vi "Follow 1D Motion Profile for Turning.vi"(4 "PID gains":T20 {"derivative time (Td, min)" format="%.3f"; "integral time (Ti, min)" format="%.3f"; "proportional gain (Kc)" format="%.3f"}, 6 "Period (s)":dbl=0.005, 7 "output range":cluster{"output high":dbl, "output low":dbl}={"output high"=1.0, "output low"=-1.0} {"output low" format="%.2f"; "output high" format="%.2f"}, 8 "Ka":dbl, 9 "Kv":dbl, 10 "Profile":T21, 11 "auton ref":T1={"Starting Pos"=0, "Defence"=enum."Chivel De Fris", "Drivetrain"={"DevStatus"={"status"=FALSE, "code"=0, "source"=""}, "Motors[]"=[], "Square Inputs"=FALSE, "Max Output"=1.0}, "State"=enum."Drive to Outerworks", "Encoder Right"={"DevStatus"={"status"=FALSE, "code"=0, "source"=""}, "EncoderIndex"=enum."Invalid", "CounterIndex"=enum."Invalid", "DistancePerCount"=1.0, "Decoding Type"=enum."4x"}, "Encoder Left"={"DevStatus"={"status"=FALSE, "code"=0, "source"=""}, "EncoderIndex"=enum."Invalid", "CounterIndex"=enum."Invalid", "DistancePerCount"=1.0, "Decoding Type"=enum."4x"}, "Line Sensor"={"DevStatus"={"status"=FALSE, "code"=0, "source"=""}, "DIO Channel"=enum."Invalid", "CntIndex"=enum."Invalid", "Normally Closed"=FALSE}, "navX"={"Interface"={"Protocol"=enum."SERIAL", "Update Rate (4Hz-60Hz)"=4, "navX Open TypeDef"=variant}, "Notify Packet"=refnum, "Loop VI Refnum"=refnum, "Ready to Close Occurrence Refnum"=refnum}, "Front Arm"={"DevStatus"={"status"=FALSE, "code"=0, "source"=""}, "Analog Channel"=enum."Invalid", "Invert Output"=FALSE}, "Start Time"=0, "State Vars"=variant} {"navX"."Interface"."Update Rate (4Hz-60Hz)" min=4 max=60 step=1}) -> ()   [LabVIEW 2016]
uses:
  <vilib>/Platform/TimedLoop/XDataNode/XDataNode.xnode
  <vilib>/Platform/TimedLoop/XDataNode/nitl_modes.ctl
  <vilib>/Platform/TimedLoop/XDataNode/XDNodeRunTimeDep.lvlib
  <vilib>/Platform/TimedLoop/XDataNode/wakeup.ctl
  <vilib>/Platform/TimedLoop/XDataNode/timing_clust.ctl
  <vilib>/addons/control/pid/NI_PID_pid.lvlib
  <vilib>/addons/control/pid/pid.llb/PID (DBL).vi
  Robot Global Data.vi
  Typedef/Motion Profile.ctl
  NavX/TypeDefs/Z900_navX_ProtocolTypeDef.ctl
  NavX/TypeDefs/Z900_navX_ActionTypeDef.ctl
  NavX/TypeDefs/Z900_navX_NotifyPacketTypeDef.ctl
  NavX/TypeDefs/Z900_navX_DeviceTypeDef.ctl
  <vilib>/Rock Robotics/SystemInterfaces/DIO/FPGA_DIOChannel.ctl
  <vilib>/Rock Robotics/SystemInterfaces/Counter/FPGA_CounterCtrSystemIndex.ctl
  <vilib>/Rock Robotics/WPI/Switch/WPI_SwitchDevRef.ctl
  <vilib>/Rock Robotics/SystemInterfaces/Encoder/FPGA_EncoderIdx.ctl
  <vilib>/Rock Robotics/WPI/Encoder/WPI_EncoderType.ctl
  <vilib>/Rock Robotics/WPI/Encoder/WPI_EncoderDevRef.ctl
  Typedef/MainStates.ctl
  <vilib>/Rock Robotics/SystemInterfaces/DIO/FPGA_DIOPWMChannel.ctl
  <vilib>/Rock Robotics/WPI/PWM/WPI_PWMDeadband.ctl
  <vilib>/Rock Robotics/WPI/MotorControl/WPI_MotorControlType.ctl
  <vilib>/Rock Robotics/WPI/MotorControl/WPI_MotorControlDeviceRef.ctl
  <vilib>/Rock Robotics/WPI/RobotDrive/WPI_RobotDriveDevRef.ctl
  Typedef/Defences.ctl
  Typedef/AutonRefType.ctl
  <vilib>/Rock Robotics/SystemInterfaces/AI/FPGA_AIChannel.ctl
  <vilib>/Rock Robotics/WPI/Potentiometer/WPI_PotentiometerDevRef.ctl
panel:
  in  "Eliminate Deadband":bool=TRUE
  out "Waveform Chart":T19(graph)
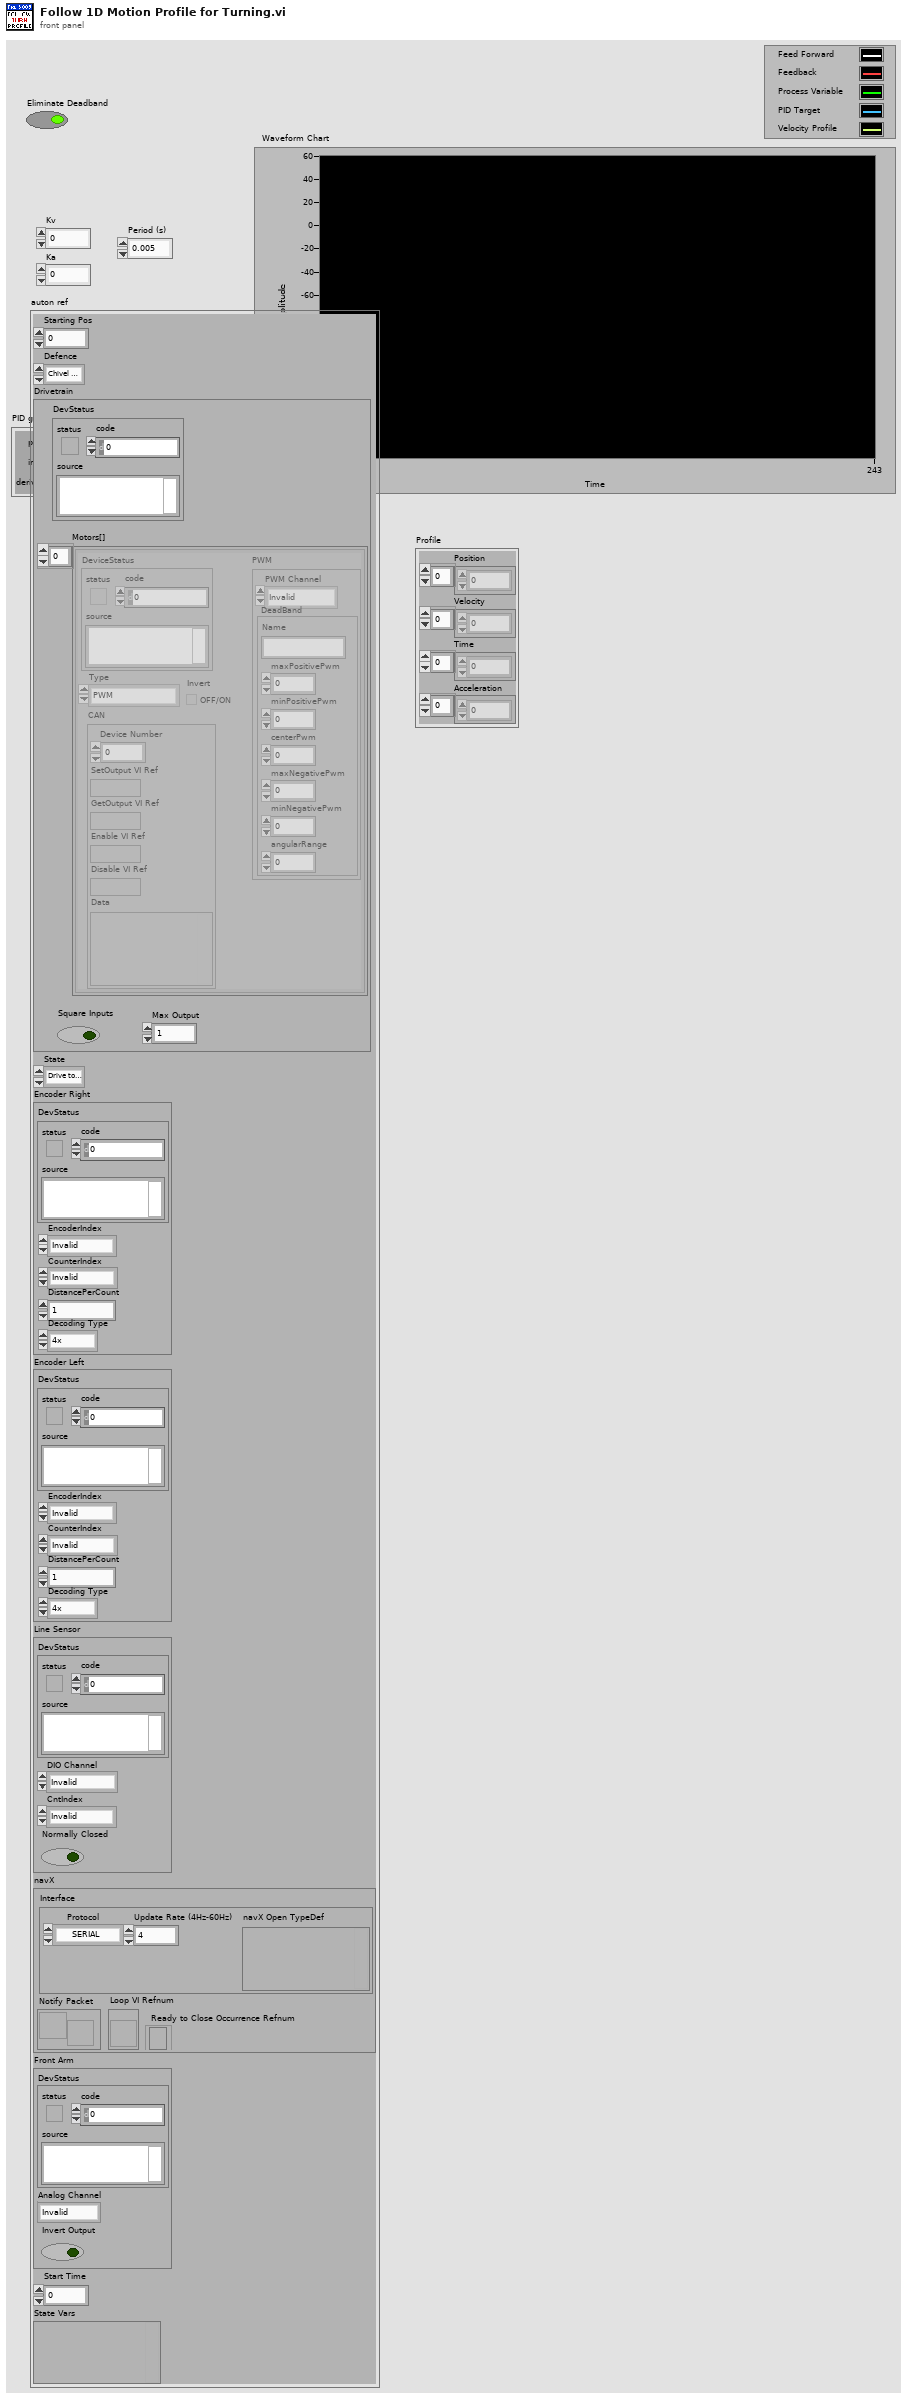
[diagram p1: front panel]
types:
  T1 = typedef "AutonRefType.ctl" = cluster{"Starting Pos":u32, "Defence":T2, "Drivetrain":T3, "State":T8, "Encoder Right":T9, "Encoder Left":T9, "Line Sensor":T13, "navX":T15, "Front Arm":T17, "Start Time":u32, "State Vars":variant}
  T2 = typedef "Defences.ctl" = enum16{"Low Bar", "Chivel De Fris", "Sally Port", "Portcullis", "Draw Bridge", "Moat", "Rough Terrain", "Ramparts", "Rock Wall"}
  T3 = typedef "WPI_RobotDriveDevRef.ctl" = cluster{"DevStatus":errorcluster, "Motors[]":T4[], "Square Inputs":bool, "Max Output":dbl}
  T4 = typedef "WPI_MotorControlDeviceRef.ctl" = cluster{"DeviceStatus":errorcluster, "Type":T5, "PWM":cluster{"PWM Channel":T6, "DeadBand":T7}, "CAN":cluster{"Device Number":u8, "SetOutput VI Ref":variant, "GetOutput VI Ref":variant, "Enable VI Ref":variant, "Disable VI Ref":variant, "Data":variant}, "Invert":bool}
  T5 = typedef "WPI_MotorControlType.ctl" = enum16{"PWM", "CAN"}
  T6 = typedef "FPGA_DIOPWMChannel.ctl" = enum8{"PWM 0", "PWM 1", "PWM 2", "PWM 3", "PWM 4", "PWM 5", "PWM 6", "PWM 7", "PWM 8", "PWM 9", "PWM MXP 0", "PWM MXP 1", "PWM MXP 2", "PWM MXP 3", "PWM MXP 4", "PWM MXP 5", "PWM MXP 6", "PWM MXP 7", "PWM MXP 8", "PWM MXP 9", "Invalid"}
  T7 = typedef "WPI_PWMDeadband.ctl" = cluster{"Name":string, "maxPositivePwm":i32, "minPositivePwm":i32, "centerPwm":i32, "maxNegativePwm":i32, "minNegativePwm":i32, "angularRange":u16}
  T8 = typedef "MainStates.ctl" = enum16{"Drive to Outerworks", "Cross Defence", "Align to Line", "Turn to Goal", "Find Position", "Find Distance", "Drive to Scoring Location", "Score Low Goal", "SquareToField", "Hit Driver Station Wall", "Drive Back to Position", "CDF", "Cleanup", "_TEST_Profile", "_TEST_TurnProfile", "_TEST_Impulse", "Error"}
  T9 = typedef "WPI_EncoderDevRef.ctl" = cluster{"DevStatus":errorcluster, "EncoderIndex":T10, "CounterIndex":T11, "DistancePerCount":dbl, "Decoding Type":T12}
  T10 = typedef "FPGA_EncoderIdx.ctl" = enum8{"Enc 0", "Enc 1", "Enc 2", "Enc 3", "Enc 4", "Enc 5", "Enc 6", "Enc 7", "Invalid"}
  T11 = typedef "FPGA_CounterCtrSystemIndex.ctl" = enum8{"Ctr 0", "Ctr 1", "Ctr 2", "Ctr 3", "Ctr 4", "Ctr 5", "Ctr 6", "Ctr 7", "Invalid"}
  T12 = typedef "WPI_EncoderType.ctl" = enum16{"1x", "2x", "4x"}
  T13 = typedef "WPI_SwitchDevRef.ctl" = cluster{"DevStatus":errorcluster, "DIO Channel":T14, "CntIndex":T11, "Normally Closed":bool}
  T14 = typedef "FPGA_DIOChannel.ctl" = enum8{"DIO 0", "DIO 1", "DIO 2", "DIO 3", "DIO 4", "DIO 5", "DIO 6", "DIO 7", "DIO 8", "DIO 9", "DIO MXP 0", "DIO MXP 1", "DIO MXP 2", "DIO MXP 3", "DIO MXP 4", "DIO MXP 5", "DIO MXP 6", "DIO MXP 7", "DIO MXP 8", "DIO MXP 9", "DIO MXP 10", "DIO MXP 11", "DIO MXP 12", "DIO MXP 13", "DIO MXP 14", "DIO MXP 15", "SPI Port CS1", "SPI Port CS2", "SPI Port CS3", "SPI Port MISO", "SPI Port MOSI", "Invalid"}
  T15 = typedef "navX Library v2.lvlib/Z900_navX_DeviceTypeDef.ctl" = cluster{"Interface":cluster{"Protocol":T16, "Update Rate (4Hz-60Hz)":u8, "navX Open TypeDef":variant}, "Notify Packet":refnum<notifier>, "Loop VI Refnum":refnum<vi>, "Ready to Close Occurrence Refnum":refnum<k4>}
  T16 = typedef "navX Library v2.lvlib/Z900_navX_ProtocolTypeDef.ctl" = enum16{"SERIAL", "I2C", "SPI"}
  T17 = typedef "WPI_PotentiometerDevRef.ctl" = cluster{"DevStatus":errorcluster, "Analog Channel":T18, "Invert Output":bool}
  T18 = typedef "FPGA_AIChannel.ctl" = enum8{"AI 0", "AI 1", "AI 2", "AI 3", "AI MXP 0", "AI MXP 1", "AI MXP 2", "AI MXP 3", "Invalid"}
  T19 = cluster{dbl, "output":dbl, dbl, dbl, "Max Velocity":dbl}
  T20 = cluster{"proportional gain (Kc)":dbl, "integral time (Ti, min)":dbl, "derivative time (Td, min)":dbl}
  T21 = typedef "Motion Profile.ctl" = cluster{"Position":dbl[], "Velocity":dbl[], "Time":dbl[], "Acceleration":dbl[]}
  T22 = cluster{"Yaw":dbl, "Roll":dbl, "Pitch":dbl, "Heading":dbl, "Fused Heading":dbl}
  T23 = typedef "XDNodeRunTimeDep.lvlib/timing_clust.ctl" = cluster{"Expected End [f-1]":u64, "Actual End [f-1]":u64, "Finished Late? [f-1]":bool, "Expected End [i-1]":u64, "Actual End [i-1]":u64, "Finished Late? [i-1]":bool, "Expected Start [i]":u64, "Actual Start [i]":u64, "Expected Start [f]":u64, "Actual Start [f]":u64, "Source Name":string, "Structure Name":string, "Period":i64, "Deadline":i64, "Offset":i64, "Start":i64, "Priority":i32, "Timeout":i32, "Mode":T24, "Wakeup Reason":T25, "Error":errorcluster, "Source Type":string, "Secondary Source Type":string, "Global End Time":u64, "Global Start Time":u64, "Frame Duration":u64, "Iteration Duration":u64, "Assigned CPU":i32, "I/O Scan Engine Mode":u32}
  T24 = typedef "XDNodeRunTimeDep.lvlib/nitl_modes.ctl" = enum32{"No Change", "Process missed periods, maintain original phase", "Discard missed periods, maintain original phase", "Process missed periods, ignore original phase", "Discard missed periods, ignore original phase"}
  T25 = typedef "XDNodeRunTimeDep.lvlib/wakeup.ctl" = enum32{"Normal", "Aborted", "Asynchronous wakeup", "Timing source error", "Timed loop error", "Timeout"}
  T26 = cluster{dbl, "output":dbl, dbl, "Angle (rads)":dbl, "Max Velocity":dbl}
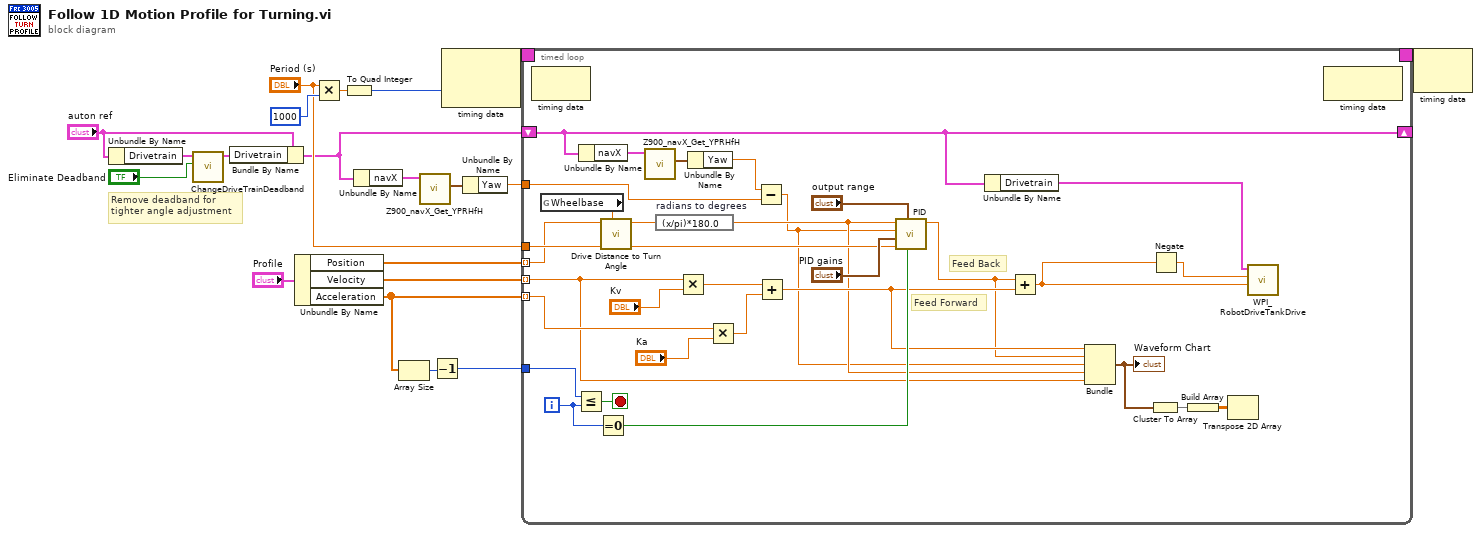
[diagram p0: block diagram]
diagram:
  # "Remove deadband for \ntighter angle adjustment"
  n1 = Unbundle By Name("auton ref") -> ("Drivetrain"=w5:T3)
  n2 = call "ChangeDriveTrainDeadband.vi"("Eliminate Deadband"="Eliminate Deadband", "Drivetrain in"=w5) -> ("Drivetrain out"=w2:T3)  [unwired: 9 in]
  n3 = Bundle By Name(cluster="auton ref", "Drivetrain"=w2) -> (w1:T1)
  n4 = Unbundle By Name("Profile") -> ("Position"=w17:dbl[], "Velocity"=w16:dbl[], "Acceleration"=w15:dbl[])
  n5 = Multiply(x="Period (s)", y=1000) -> (x*y=w11:dbl)
  n6 = To Quad Integer(1:w11) -> (0:w10:i64)
  n7 = Unbundle By Name(w1) -> ("navX"=w7:T15)
  n8 = Array Size(array=w15) -> (size(s)=w14:i32)
  n9 = call "Z900_navX_Get_YPRHfH.vi"("navX Device"=w7) -> ("YRPHfH"=w8:T22)  [unwired: 7 in, 3 out]
  n10 = Decrement(x=w14) -> (x-1=w13:i32)
  n11 = node-c288(w10) -> (w20:T23)  [unwired: 1 in]
  n12 = Unbundle By Name(w8) -> ("Yaw"=w6:dbl)
  n13 = timed-loop {
    timing: w20 -> [_]
    timing-out: [_] -> w19
    tunnel: w17 -> [w37] mode=indexing
    tunnel: w16 -> [w36] mode=indexing
    tunnel: w15 -> [w40] mode=indexing
    tunnel: w13 -> [w51]
    tunnel: "Period (s)" -> [w43]
    shift-right: [w35] -> _
    shift-left: w1 -> [w35]
    tunnel: w6 -> [w27]
    i -> [w42]
    stop <- w50 stop-if-true
    # "Feed Back"
    # "Feed Forward"
    n14 = node-c288() -> ()  [unwired: 1 in, 1 out]
    n15 = global read "Robot Global Data.vi" "Wheelbase"() -> (w30:dbl)
    n16 = Less Or Equal?(x=w51, y=w42) -> (x <= y?=w50:bool)
    n17 = Unbundle By Name(w35) -> ("navX"=w34:T15)
    n18 = Equal To 0?(x=w42) -> (x = 0?=w41:bool)
    n19 = call "Drive Distance to Turn Angle.vi"("Wheelbase (in)"=w30, "Distance (in)"=w37) -> ("Angle (rads)"=w31:dbl)  [unwired: 7 in]
    n20 = call "Z900_navX_Get_YPRHfH.vi"("navX Device"=w34) -> ("YRPHfH"=w33:T22)  [unwired: 7 in, 3 out]
    n21 = expression code="(x/pi)*180.0" "radians to degrees"(w31) -> (w29:dbl)
    n22 = Multiply(x=w36, y="Kv") -> (x*y=w47:dbl)
    n23 = Unbundle By Name(w33) -> ("Yaw"=w32:dbl)
    n24 = Multiply(x=w40, y="Ka") -> (x*y=w46:dbl)
    n25 = Subtract(x=w32, y=w27) -> (x-y=w28:dbl)
    n26 = Add(x=w47, y=w46) -> (x+y=w39:dbl)
    n27 = call-poly <vilib>:"PID.vi"("reinitialize? (F)"=w41, "output range"="output range", "dt (s)"=w43, "PID gains"="PID gains", "process variable"=w28, "setpoint"=w29) -> ("output"=w38:dbl)  [unwired: 4 in, 1 out]
    n28 = Unbundle By Name(w35) -> ("Drivetrain"=w21:T3)
    n29 = Add(x=w38, y=w39) -> (x+y=w26:dbl)
    n30 = Bundle(w39, "output"=w38, w28, "Angle (rads)"=w29, "Max Velocity"=w36) -> (w22:T26)  [unwired: 1 in]
    "Waveform Chart" <- w22
    n31 = Cluster To Array(cluster=w22) -> (array=w24:dbl[])
    n32 = Negate(x=w26) -> (-x=w25:dbl)
    n33 = Build Array(w24) -> (w23:dbl[][])
    n34 = Transpose 2D Array(2D array=w23) -> ()  [unwired: 1 out]
    n35 = call <vilib>:"WPI_RobotDriveTankDrive.vi"("Right axis value"=w26, "Left axis value"=w25, "RobotDriveDevRef"=w21) -> ()  [unwired: 6 in, 3 out]
    n36 = node-c288() -> ()  [unwired: 1 in, 1 out]
  }
  n37 = node-c288(w19) -> ()  [unwired: 1 out]
